vi "Display Wf(SubVI).vi"(11 "NavData Out":T2) -> (1 "vx (cm/s)?":sgl, 2 "altitude (cm)":u32, 3 "Cluster":T1, 4 "vy (cm/s)?":sgl, 5 "battery percentage":u32)   [LabVIEW 2014]
uses:
  <vilib>/LVH/AR Drone Toolkit/Decode NavData/Typedefs/NavData Demo.ctl
  <vilib>/LVH/AR Drone Toolkit/AR Drone.lvlib
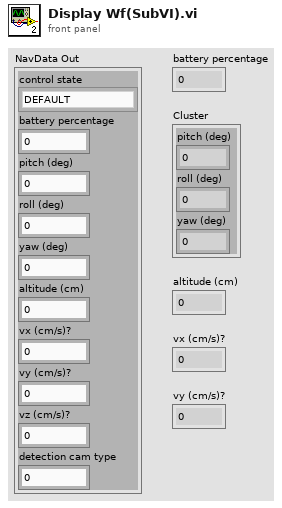
[diagram p1: front panel]
types:
  T1 = cluster{"pitch (deg)":sgl, "roll (deg)":sgl, "yaw (deg)":sgl}
  T2 = typedef "AR Drone.lvlib/NavData Demo.ctl" = cluster{"control state":enum32{"DEFAULT", "INIT", "LANDING", "FLYING", "HOVERING", "TEST", "TRANS_TAKEOFF", "TRANS_GOTOFIX", "TRANS_LANDING"}, "battery percentage":u32, "pitch (deg)":sgl, "roll (deg)":sgl, "yaw (deg)":sgl, "altitude (cm)":u32, "vx (cm/s)?":sgl, "vy (cm/s)?":sgl, "vz (cm/s)?":sgl, "detection cam type":u32}
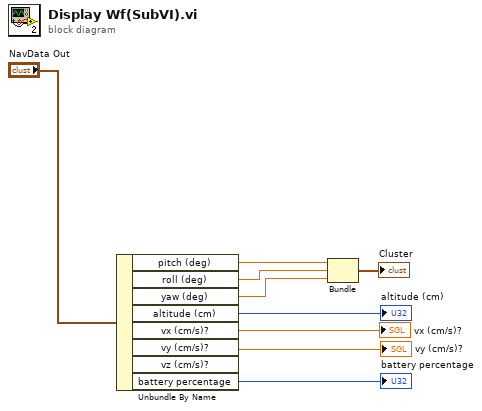
[diagram p0: block diagram]
diagram:
  n1 = Unbundle By Name("NavData Out") -> ("pitch (deg)"=w4:sgl, "roll (deg)"=w1:sgl, "yaw (deg)"=w2:sgl, "altitude (cm)"=→"altitude (cm)":u32, "vx (cm/s)?"=→"vx (cm/s)?":sgl, "vy (cm/s)?"=→"vy (cm/s)?":sgl, "battery percentage"=→"battery percentage":u32)  [unwired: 1 out]
  n2 = Bundle("pitch (deg)"=w4, "roll (deg)"=w1, "yaw (deg)"=w2) -> (→"Cluster":T1)  [unwired: 1 in]
